vi "salMain2.vi"() -> ()   [LabVIEW 2012]
uses:
  FileSelector/FileSelector.lvclass
  IDLFile/IDLFile.lvclass
panel:
  out "error out":errorcluster
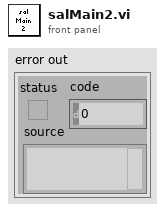
[diagram p1: front panel]
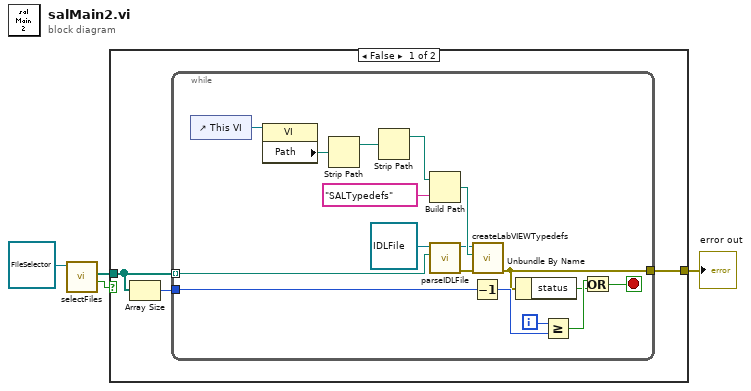
[diagram p0: block diagram]
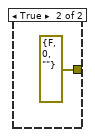
[diagram p2: hidden frame]
diagram:
  n1 = call "selectFiles.vi"("FileSelector in"=refnum<class "FileSelector.lvclass"> refnum) -> ("cancelledIsTrue"=w2:bool, "selected paths"=w1:path[])  [unwired: 7 in, 2 out]
  n2 = case shown="False" w2 {
    tunnel: [w7 errorcluster {"status"=FALSE, "code"=0, "source"=""} ("error out")] -> w3
    tunnel: w1 -> [w5 _]
    frame False {
      n3 = Array Size(array=w5) -> (size(s)=w6:i32)
      n4 = while {
        tunnel: [w11] -> w7
        tunnel: w5 -> [w8] mode=indexing
        tunnel: w6 -> [w13]
        i -> [w14]
        stop <- w9 stop-if-true
        n5 = control-ref of="This VI"() -> (w24:refnum<vi>)
        n6 = property class="VI"(reference=w24) -> ("Path"=w23:path)  [unwired: 1 in, 2 out]
        n7 = Strip Path(path=w23) -> (stripped path=w21:path)  [unwired: 1 out]
        n8 = Strip Path(path=w21) -> (stripped path=w19:path)  [unwired: 1 out]
        n9 = Build Path(base path=w19, name or relative path="SALTypedefs") -> (appended path=w18:path)
        n10 = call "parseIDLFile.vi"("idlFilepath"=w8, "IDLFile in"=refnum<class "IDLFile.lvclass"> refnum ("IDLParser in")) -> ("error out"=w16:errorcluster, "IDLFile out"=w17:refnum<class "IDLFile.lvclass">)  [unwired: 8 in]
        n11 = Decrement(x=w13) -> (x-1=w15:i32)
        n12 = call "createLabVIEWTypedefs.vi"("error in (no error)"=w16, "targetBasePath"=w18, "IDLFile in"=w17) -> ("error out"=w11:errorcluster)  [unwired: 7 in, 1 out]
        n13 = Unbundle By Name(w11) -> ("status"=w10:bool)
        n14 = Greater Or Equal?(x=w14, y=w15) -> (x >= y?=w12:bool)
        n15 = Or(x=w12, y=w10) -> (x .or. y?=w9:bool)
      }
    }
    frame True {
    }
  }
  "error out" <- w3
